vi "alarm.vi"() -> ()   [LabVIEW 2015]
panel:
  in  "Cluster 2":T1={"SCAN BAR CODE"=16318208, "BAR CODE OK"=6618880, "BAR CODE NG"=16711680, "BAR CODE ALREADY RUN"=16711680, "RESET PUSH BUTTON PRESSED"=16711680, "E.STOP PUSH BUTTON PRESSED"=16711680, "MAIN PRESSURE FAIL"=16711680, "CLAMP HOME RS FAIL"=16711680, "CLAMP END RS FAIL "=16711680, "PART NOT PRESENCE "=16711680, "VANT CAP 1 NOT PRESENCE"=16711680, "VANT CAP 2 NOT PRESENCE"=16711680, "JIG NOT CONNECTED"=16711680, "\tMAIN PRESSURE FAIL 2"=16711680, "VANT CAP 1,2 NOT PRESENCE"=16711680, "BAR CODE NOT SCAN"=16711680, "CAMERA ERROR "=16711680, "MACHINE SIDE DOOR OPEN"=16711680, "MACHINE READY FOR NEXT CYCLE"=6618880, "ALL LED ON "=16318208, "\tALL LED LOW CURRENT NG"=16711680, "\tALL LED HIGH CURRENT NG"=16711680, "HIGH BEAM LOW CURRENT NG"=16711680, "HIGH BEAM HIGH CURRENT NG"=16711680, "HIGH BEAM IMAGE NG"=16711680, "POSITION BEAM ON "=16318208, "POSITION BEAM LOW CURRENT NG"=16711680, "POSITION BEAM HIGH CURRENT NG"=16711680, "POSITION BEAM IMAGE NG"=16711680, "LOW BEAM ON"=16318208, "LOW BEAM LOW CURRENT NG"=16711680, "LOW BEAM HIGH CURRENT NG"=16711680, "LOW BEAM IMAGE NG"=16711680, "PART OK REMOVE PART "=6618880, "HIGH BEAM VOLTAGE HIGH"=16711680, "\tLOW BEAM VOLTAGE HIGH"=16711680, "HIGH BEAM ON"=16318208, "PATRAN ADJ. TIME OVER"=16711680, "HIGH BEAM LUX NG "=16711680, "HIGH BEAM LUX NG 2"=16711680, "LOW BEAM IMAGE NG"=16711680, "LOW BEAM IMAGE NG 2"=16711680, "POSITION IMAGE NG"=16711680, "POSITION IMAGE NG 2"=16711680}
  out "Array":string[](array[string])
  out "Cluster":T1={"SCAN BAR CODE"=16318208, "BAR CODE OK"=6618880, "BAR CODE NG"=16711680, "BAR CODE ALREADY RUN"=16711680, "RESET PUSH BUTTON PRESSED"=16711680, "E.STOP PUSH BUTTON PRESSED"=16711680, "MAIN PRESSURE FAIL"=16711680, "CLAMP HOME RS FAIL"=16711680, "CLAMP END RS FAIL "=16711680, "PART NOT PRESENCE "=16711680, "VANT CAP 1 NOT PRESENCE"=16711680, "VANT CAP 2 NOT PRESENCE"=16711680, "JIG NOT CONNECTED"=16711680, "\tMAIN PRESSURE FAIL 2"=16711680, "VANT CAP 1,2 NOT PRESENCE"=16711680, "BAR CODE NOT SCAN"=16711680, "CAMERA ERROR "=16711680, "MACHINE SIDE DOOR OPEN"=16711680, "MACHINE READY FOR NEXT CYCLE"=6618880, "ALL LED ON "=16318208, "\tALL LED LOW CURRENT NG"=16711680, "\tALL LED HIGH CURRENT NG"=16711680, "HIGH BEAM LOW CURRENT NG"=16711680, "HIGH BEAM HIGH CURRENT NG"=16711680, "HIGH BEAM IMAGE NG"=16711680, "POSITION BEAM ON "=16318208, "POSITION BEAM LOW CURRENT NG"=16711680, "POSITION BEAM HIGH CURRENT NG"=16711680, "POSITION BEAM IMAGE NG"=16711680, "LOW BEAM ON"=16318208, "LOW BEAM LOW CURRENT NG"=16711680, "LOW BEAM HIGH CURRENT NG"=16711680, "LOW BEAM IMAGE NG"=16711680, "PART OK REMOVE PART "=6618880, "HIGH BEAM VOLTAGE HIGH"=16711680, "\tLOW BEAM VOLTAGE HIGH"=16711680, "HIGH BEAM ON"=16318208, "PATRAN ADJ. TIME OVER"=16711680, "HIGH BEAM LUX NG "=16711680, "HIGH BEAM LUX NG 2"=16711680, "LOW BEAM IMAGE NG"=16711680, "LOW BEAM IMAGE NG 2"=16711680, "POSITION IMAGE NG"=16711680, "POSITION IMAGE NG 2"=16711680}
  # "1\tM69\tSCAN BAR CODE\n2\tM70\tBAR CODE OK\n3\tM71\tBAR CODE NG\n4\tM72\tBAR CODE ALREADY RUN\n5\tM100\tRESET PUSH BUTTON PRESSED\n6\tM101\tE.STOP PUSH BUTTON PRESSED\n7\tM102\tMAIN PRESSURE FAIL \n8\tM103\tCLAMP HOME RS FAIL\n9\tM104\tCLAMP END RS FAIL \n10\tM105\tPART NOT PRESENCE \n11\tM106\tVANT CAP 1 NOT PRESENCE\n12\tM107\tVANT CAP 2 NOT PRESENCE\n13\tM108\tJIG NOT CONNECTED\n14\tM109\tMAIN PRESSURE FAIL\n15\tM110\tVANT CAP 1, 2 NOT PRESENCE\n16\tM111\tBAR CODE NOT SCAN \n17\tM112\tCAMERA ERROR \n18\tM113\tMACHINE SIDE DOOR OPEN\n19\tM150\tMACHINE READY FOR NEXT CYCLE\n20\tM153\tALL LED ON \n21\tM157\tALL LED LOW CURRENT NG\n22\tM158\tALL LED HIGH CURRENT NG\n23\tM163\tHIGH BEAM LOW CURRENT NG\n24\tM164\tHIGH BEAM HIGH CURRENT NG\n25\tM168\tHIGH BEAM IMAGE NG \n26\tM172\tPOSITION BEAM ON \n27\tM175\tPOSITION BEAM LOW CURRENT NG\n28\tM176\tPOSITION BEAM HIGH CURRENT NG\n29\tM180\tPOSITION BEAM IMAGE NG \n30\tM181\tLOW BEAM ON \n31\tM184\tLOW BEAM LOW CURRENT NG\n32\tM185\tLOW BEAM HIGH CURRENT NG\n33\tM189\tLOW BEAM IMAGE NG \n34\tM192\tPART OK REMOVE PART \n35\tM193\tHIGH BEAM VOLTAGE HIGH \n36\tM194\tLOW BEAM VOLTAGE HIGH\n37\tM196\tHIGH BEAM ON\n38\tM215\tPATRAN ADJ. TIME OVER\n39\tM221\tHIGH BEAM LUX NG \n40\tM222\tHIGH BEAM LUX NG\n41\tM224\tLOW BEAM IMAGE NG\n42\tM225\tLOW BEAM IMAGE NG\n43\tM227\tPOSITION IMAGE NG\n44\tM228\tPOSITION IMAGE NG"
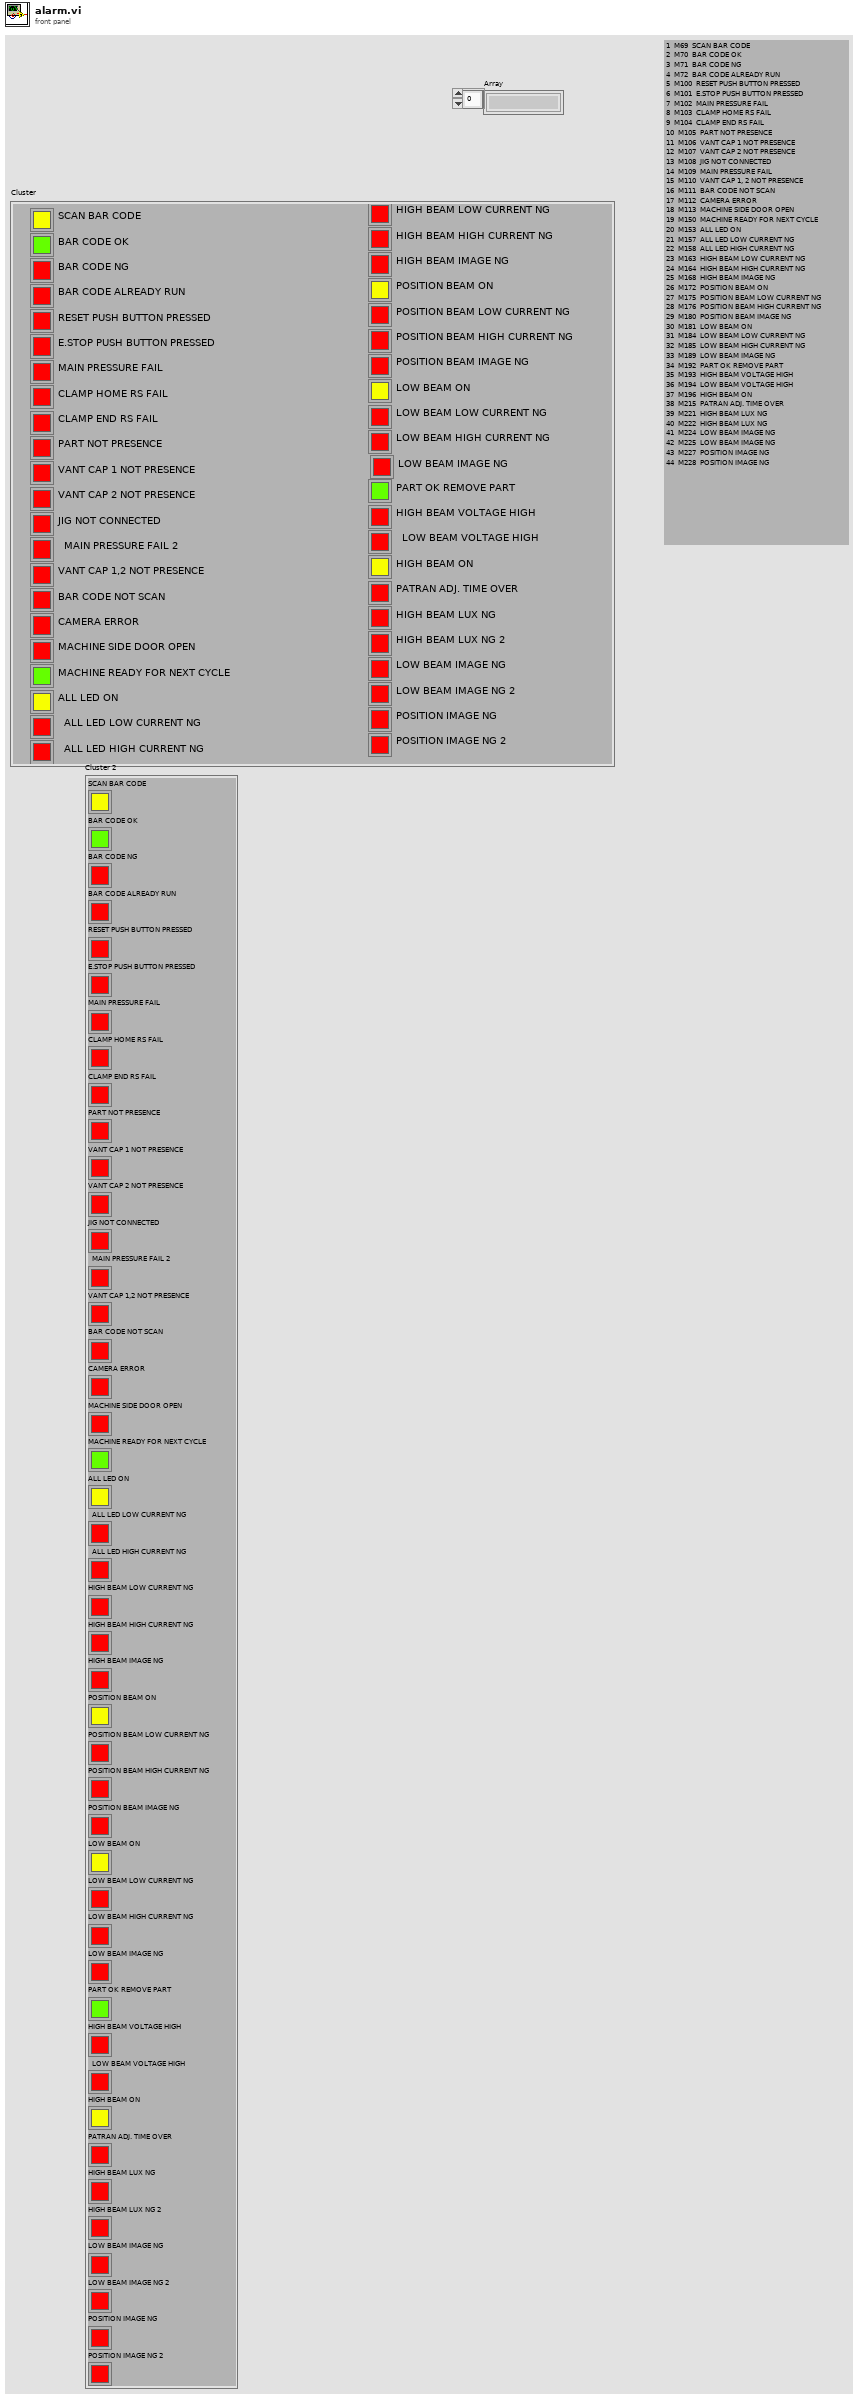
[diagram p1: front panel]
types:
  T1 = cluster{"SCAN BAR CODE":u32, "BAR CODE OK":u32, "BAR CODE NG":u32, "BAR CODE ALREADY RUN":u32, "RESET PUSH BUTTON PRESSED":u32, "E.STOP PUSH BUTTON PRESSED":u32, "MAIN PRESSURE FAIL":u32, "CLAMP HOME RS FAIL":u32, "CLAMP END RS FAIL ":u32, "PART NOT PRESENCE ":u32, "VANT CAP 1 NOT PRESENCE":u32, "VANT CAP 2 NOT PRESENCE":u32, "JIG NOT CONNECTED":u32, "\tMAIN PRESSURE FAIL 2":u32, "VANT CAP 1,2 NOT PRESENCE":u32, "BAR CODE NOT SCAN":u32, "CAMERA ERROR ":u32, "MACHINE SIDE DOOR OPEN":u32, "MACHINE READY FOR NEXT CYCLE":u32, "ALL LED ON ":u32, "\tALL LED LOW CURRENT NG":u32, "\tALL LED HIGH CURRENT NG":u32, "HIGH BEAM LOW CURRENT NG":u32, "HIGH BEAM HIGH CURRENT NG":u32, "HIGH BEAM IMAGE NG":u32, "POSITION BEAM ON ":u32, "POSITION BEAM LOW CURRENT NG":u32, "POSITION BEAM HIGH CURRENT NG":u32, "POSITION BEAM IMAGE NG":u32, "LOW BEAM ON":u32, "LOW BEAM LOW CURRENT NG":u32, "LOW BEAM HIGH CURRENT NG":u32, "LOW BEAM IMAGE NG":u32, "PART OK REMOVE PART ":u32, "HIGH BEAM VOLTAGE HIGH":u32, "\tLOW BEAM VOLTAGE HIGH":u32, "HIGH BEAM ON":u32, "PATRAN ADJ. TIME OVER":u32, "HIGH BEAM LUX NG ":u32, "HIGH BEAM LUX NG 2":u32, "LOW BEAM IMAGE NG":u32, "LOW BEAM IMAGE NG 2":u32, "POSITION IMAGE NG":u32, "POSITION IMAGE NG 2":u32}
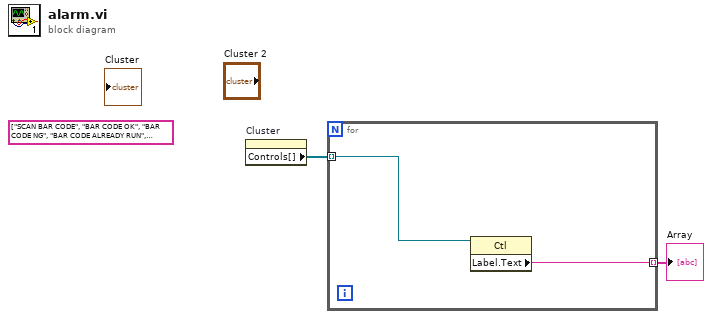
[diagram p0: block diagram]
diagram:
  (unwired) string[] ["SCAN BAR CODE", "BAR CODE OK", "BAR CODE NG", "BAR CODE ALREADY RUN", "RESET PUSH BUTTON PRESSED", "E.STOP PUSH BUTTON PRESSED", "MAIN PRESSURE FAIL", "CLAMP HOME RS FAIL", "CLAMP END RS FAIL ", "PART NOT PRESENCE ", "VANT CAP 1 NOT PRESENCE", "VANT CAP 2 NOT PRESENCE", "JIG NOT CONNECTED", "\tMAIN PRESSURE FAIL 2", "VANT CAP 1,2 NOT PRESENCE", "BAR CODE NOT SCAN", "CAMERA ERROR ", "MACHINE SIDE DOOR OPEN", "MACHINE READY FOR NEXT CYCLE", "ALL LED ON ", "\tALL LED LOW CURRENT NG", "\tALL LED HIGH CURRENT NG", "HIGH BEAM LOW CURRENT NG", "HIGH BEAM HIGH CURRENT NG", "HIGH BEAM IMAGE NG", "POSITION BEAM ON ", "POSITION BEAM LOW CURRENT NG", "POSITION BEAM HIGH CURRENT NG", "POSITION BEAM IMAGE NG", "LOW BEAM ON", "LOW BEAM LOW CURRENT NG", "LOW BEAM HIGH CURRENT NG", "LOW BEAM IMAGE NG", "PART OK REMOVE PART ", "HIGH BEAM VOLTAGE HIGH", "\tLOW BEAM VOLTAGE HIGH", "HIGH BEAM ON", "PATRAN ADJ. TIME OVER", "HIGH BEAM LUX NG ", "HIGH BEAM LUX NG 2", "LOW BEAM IMAGE NG", "LOW BEAM IMAGE NG 2", "POSITION IMAGE NG", "POSITION IMAGE NG 2"] ("Array 2")
  n1 = property on="Cluster" class="Clust (strict)"() -> ("Controls[]"=w2:refnum<vi>[])  [unwired: 2 in, 2 out]
  n2 = for {
    tunnel: w2 -> [w4] mode=indexing
    tunnel: [w3] -> w1 mode=indexing
    n3 = property class="Ctl"(reference=w4) -> ("Label.Text"=w3:string)  [unwired: 1 in, 2 out]
  }
  "Array" <- w1
